vi "IStageMaxSpeed.vi"(2 "XYSpeed":dbl=12000.0, 3 "PRIORLib.IStageIn":refnum<k7>) -> (0 "error out":errorcluster, 1 "PRIORLib.IStageOut":refnum<k7>)   [LabVIEW 2011]
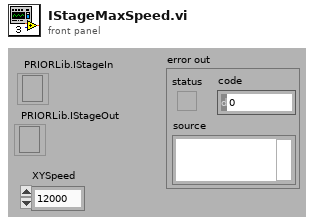
[diagram p1: front panel]
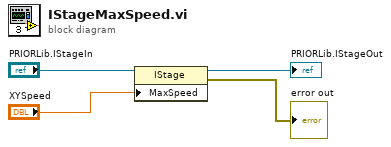
[diagram p0: block diagram]
diagram:
  n1 = property class="IStage"(reference="PRIORLib.IStageIn", "MaxSpeed"="XYSpeed") -> (reference out=→"PRIORLib.IStageOut":refnum<k7>, error out=→"error out":errorcluster)  [unwired: 1 in]
